vi "fifo configure (host).vi"(8 "error in":errorcluster, 11 "niUsrpRio Session (in)":T1 {"Daughterboard Clock Rate" format="%#.3pHz"; "FPGA Data Clock Rate" format="%#.3pHz"; "Data Clock Rate" format="%#.3pHz"; "Characterization Data"."Frequencies [Hz]" format="%#_6p"; "EEPROM Characterization Header"."Pointer to Device Data Header" format="%x"; "EEPROM Characterization Header"."Checksum" format="%x"; "Device Data Header"."Pointer to Characterization Data" format="%x"; "Device Data Header"."Checksum" format="%x"; "EEPROM Header"."Pointer to User Header" format="%x"; "EEPROM Header"."Pointer to Factory Header" format="%x"; "EEPROM Header"."Product Code" format="%x"; "EEPROM Header"."Checksum" format="%x"}) -> (0 "error out":errorcluster, 3 "niUsrpRio Session (out)":T1 {"Daughterboard Clock Rate" format="%#.3pHz"; "FPGA Data Clock Rate" format="%#.3pHz"; "Data Clock Rate" format="%#.3pHz"; "Characterization Data"."Frequencies [Hz]" format="%#_6p"; "EEPROM Characterization Header"."Pointer to Device Data Header" format="%x"; "EEPROM Characterization Header"."Checksum" format="%x"; "Device Data Header"."Pointer to Characterization Data" format="%x"; "Device Data Header"."Checksum" format="%x"; "EEPROM Header"."Pointer to User Header" format="%x"; "EEPROM Header"."Pointer to Factory Header" format="%x"; "EEPROM Header"."Product Code" format="%x"; "EEPROM Header"."Checksum" format="%x"})   [LabVIEW 2020]
uses:
  <instrlib>/niUsrpRio/Config/v1/Host/Public/niUsrpRio Session.ctl
  <instrlib>/_niInstr/Register Bus/v0/Host/Public/Register Bus Session.ctl
  <instrlib>/_niInstr/Register Bus/v0/Host/Private/Session Data.ctl
  <instrlib>/niUsrpRio/Config/v1/Host/Private/DB Queue Reference.ctl
  <instrlib>/niUsrpRio/Config/v1/Host/Private/Daughterboard Data.ctl
  <instrlib>/niUsrpRio/Config/v1/Host/Private/ATR state data.ctl
  <instrlib>/niUsrpRio/Config/v1/Host/Private/Antenna Configuration.ctl
  <instrlib>/niUsrpRio/Config/v1/Host/Private/CPLD Power Mode.ctl
  <instrlib>/niUsrpRio/Config/v1/Host/Public/EEPROM Header.ctl
  <instrlib>/niUsrpRio/Config/v1/Host/Public/EEPROM Device Data Header.ctl
  <instrlib>/niUsrpRio/Config/v1/Host/Public/EEPROM Characterization Header.ctl
  <instrlib>/niUsrpRio/Config/v1/Host/Public/Characterization Data.ctl
  <instrlib>/niUsrpRio/Config/v1/Host/Public/IQ Imbalance.ctl
  Host/SubVIs/Streaming Xvcr FPGA Ref.ctl
  <vilib>/Utility/error.llb/Error Cluster From Error Code.vi
  <vilib>/rvi/interface/common/niFpgaWaitOnOcc.vi
  <vilib>/rvi/interface/nirviMethod/nirviMethod.xnode
  <vilib>/FPGAPlugInAG/Dynamic/niLvFpga_ConfigureFifo_Dynamic.vi
  <vilib>/rvi/errors/niLvFpgaMergeErrorWithErrorCode.vi
  <vilib>/FPGAPlugInAG/Dynamic/niLvFpga_StopFifo_Dynamic.vi
  <vilib>/FPGAPlugInAG/Dynamic/niLvFpga_StartFifo_Dynamic.vi
  <instrlib>/_niInstr/Register Bus/v0/Host/niInstr Register Bus v0 Host.lvlib
  <instrlib>/niUsrpRio/Config/v1/Host/niUsrpRio Config v1 Host.lvlib
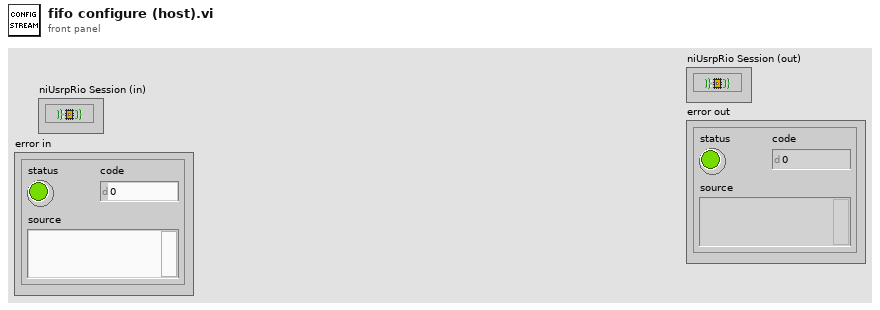
[diagram p1: front panel]
types:
  T1 = typedef "niUsrpRio Config v1 Host.lvlib/niUsrpRio Session.ctl" = cluster{"FPGA Interface":refnum<k20>, "RIO Interface Number":u32, "Data Clock Rate":u32, "FPGA Data Clock Rate":u32, "Global Settings Register Bus":T2, "Radio 0 Settings Register Bus":T2, "Radio 1 Settings Register Bus":T2, "Radio Settings Bus Semaphore":T3, "DB Queues":T4[], "Characterization Data Valid?":bool, "EEPROM Header":T5, "Device Data Header":T6, "EEPROM Characterization Header":T7, "Characterization Data":T8[], "FPGA Current Version":u32, "FPGA Oldest Compatible Version":u32, "Fixed Logic Current Version":u32, "Fixed Logic Oldest Compatible Version":u32, "FPGA Radio Settings Bus Current Version":u32, "FPGA Radio Settings Bus Oldest Compatible Version":u32, "FPGA Board Config Current Version":u32, "FPGA Board Config Oldest Compatible Version":u32, "Daughterboard Clock Rate":u32, "daughterboard configuration session handles":u64[]}
  T2 = typedef "niInstr Register Bus v0 Host.lvlib/Register Bus Session.ctl" = refnum<queue>
  T3 = typedef "Semaphore RefNum" = refnum<k1>
  T4 = typedef "niUsrpRio Config v1 Host.lvlib/DB Queue Reference.ctl" = refnum<queue>
  T5 = typedef "niUsrpRio Config v1 Host.lvlib/EEPROM Header.ctl" = cluster{"Checksum":u32, "Product Code":u16, "Hardware Current Version":u16, "Hardware Oldest Compatible Version":u16, "EEPROM Map Current Version":u16, "EEPROM Map Oldest Compatible Version":u16, "User Password":string, "Pointer to Factory Header":u32, "Pointer to User Header":u32, "Recommended Interval":u16, "Number of Reserved Bytes":i32, "Number of Daughterboards":u8, "Daughterboard IDs":u16[], "Daughterboard Serial Numbers":string[]}
  T6 = typedef "niUsrpRio Config v1 Host.lvlib/EEPROM Device Data Header.ctl" = cluster{"Checksum":u32, "Number of Channels":u8, "Number of Gain Settings":u16[], "Pointer to Characterization Data":u32[], "Number of Reserved Bytes":i32, "Number of Frequencies":u16[]}
  T7 = typedef "niUsrpRio Config v1 Host.lvlib/EEPROM Characterization Header.ctl" = cluster{"Checksum":u32, "Date":timestamp, "Temperature":sgl, "Misc. Info":string, "Pointer to Device Data Header":u32, "Number of Reserved Bytes":i32}
  T8 = typedef "niUsrpRio Config v1 Host.lvlib/Characterization Data.ctl" = cluster{"Gains[dB]":dbl[], "Frequencies [Hz]":dbl[], "IQ Imbalance Table":T9[], "Measured Gains[dB]":dbl[][]}
  T9 = typedef "niUsrpRio Config v1 Host.lvlib/IQ Imbalance.ctl" = cluster{"Gain Imbalance [linear]":dbl, "Phase Imbalance [radians]":dbl, "Offset":cdb}
  T10 = typedef "Streaming Xvcr FPGA Ref.ctl" = refnum<k20>
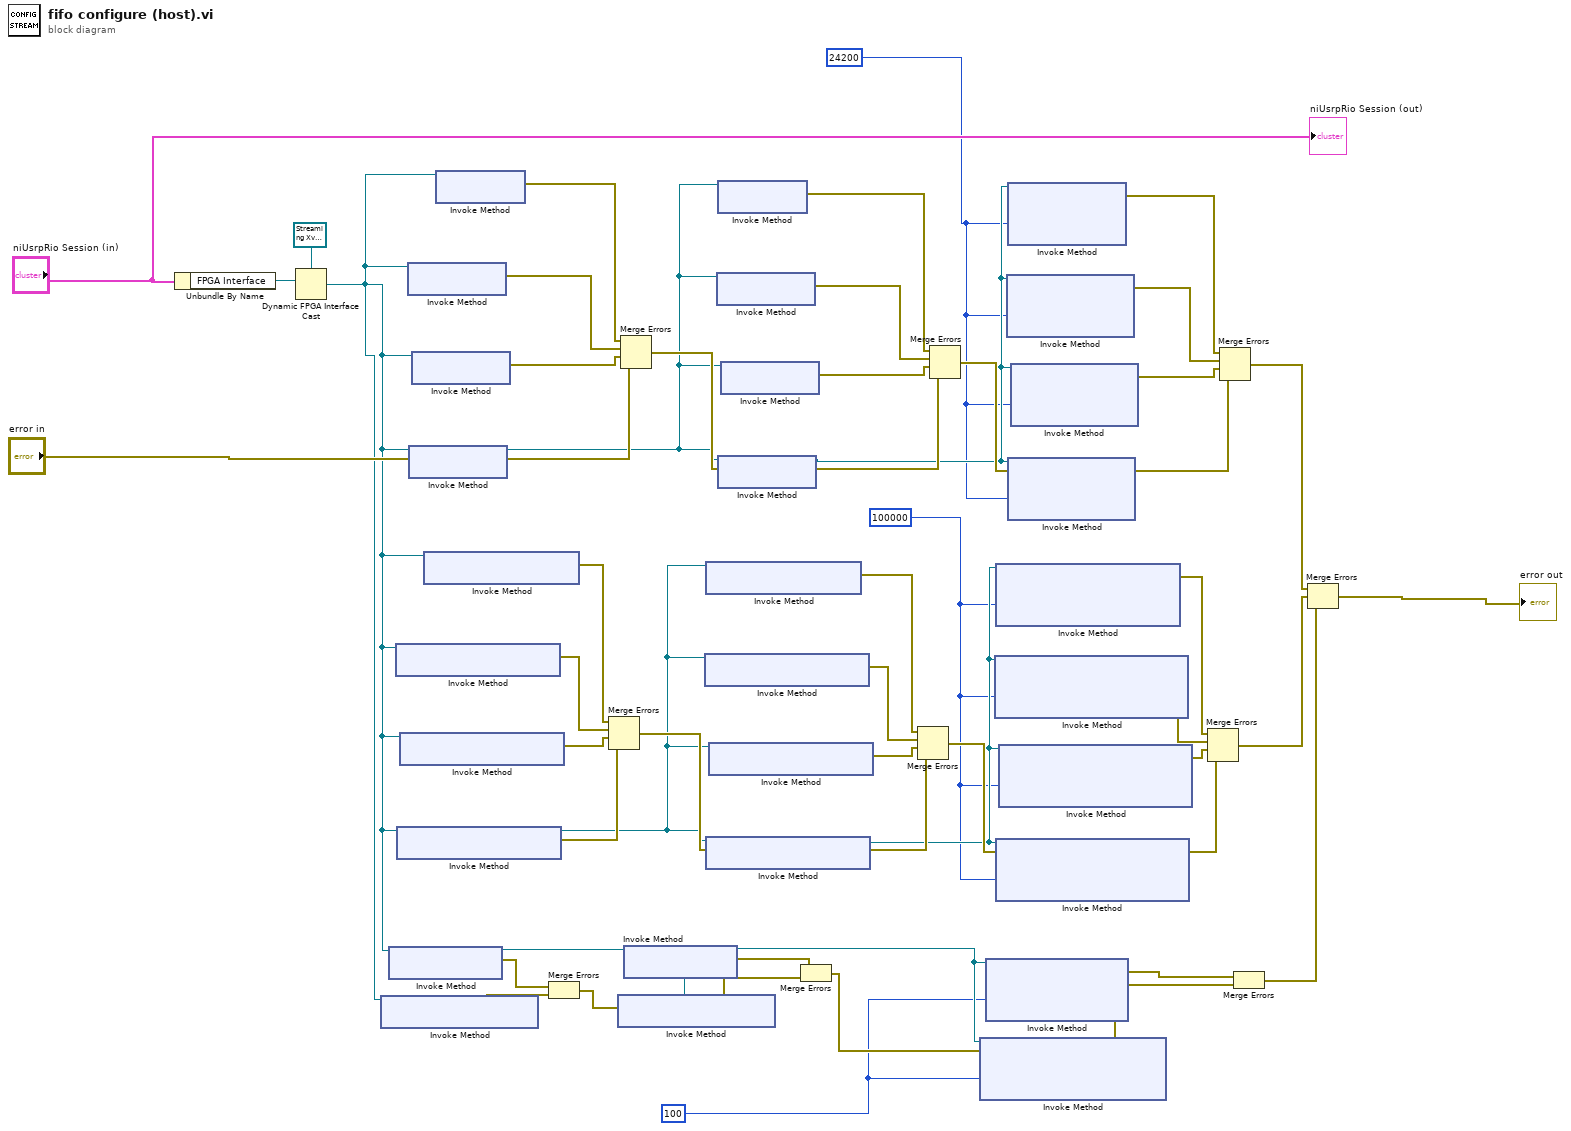
[diagram p0: block diagram]
diagram:
  w1 = u32 100000 ("Requested Depth")
  w2 = u32 24200 ("Requested Depth")
  w3 = u32 100 ("Requested Depth")
  n1 = Unbundle By Name("niUsrpRio Session (in)") -> ("FPGA Interface"=w53:refnum<k20>)
  n2 = Dynamic FPGA Interface Cast(Session In=T10 refnum ("Type"), Type=w53) -> (Session Out=w10:T10)
  n3 = xnode "Invoke Method"("FPGA VI Reference In"=w10) -> ("error out"=w15:errorcluster)  [unwired: 1 in, 1 out]
  n4 = xnode "Invoke Method"("FPGA VI Reference In"=w10) -> ("FPGA VI Reference Out"=w9:T10, "error out"=w16:errorcluster)  [unwired: 1 in]
  n5 = xnode "Invoke Method"("FPGA VI Reference In"=w10) -> ("error out"=w31:errorcluster)  [unwired: 1 in, 1 out]
  n6 = xnode "Invoke Method"("FPGA VI Reference In"=w10) -> ("FPGA VI Reference Out"=w19:T10, "error out"=w29:errorcluster)  [unwired: 1 in]
  n7 = xnode "Invoke Method"("FPGA VI Reference In"=w10) -> ("error out"=w30:errorcluster)  [unwired: 1 in, 1 out]
  n8 = xnode "Invoke Method"("FPGA VI Reference In"=w10) -> ("error out"=w50:errorcluster)  [unwired: 1 in, 1 out]
  n9 = xnode "Invoke Method"("FPGA VI Reference In"=w10, "error in"="error in") -> ("FPGA VI Reference Out"=w38:T10, "error out"=w48:errorcluster)
  n10 = xnode "Invoke Method"("FPGA VI Reference In"=w10) -> ("error out"=w49:errorcluster)  [unwired: 1 in, 1 out]
  n11 = xnode "Invoke Method"("FPGA VI Reference In"=w10) -> ("error out"=w32:errorcluster)  [unwired: 1 in, 1 out]
  n12 = xnode "Invoke Method"("FPGA VI Reference In"=w10) -> ("error out"=w51:errorcluster)  [unwired: 1 in, 1 out]
  n13 = Merge Errors(w16, w15) -> (w7:errorcluster)
  n14 = Merge Errors(w32, w31, w30, w29) -> (w20:errorcluster)
  n15 = xnode "Invoke Method"("FPGA VI Reference In"=w9, "error in"=w7) -> ("error out"=w13:errorcluster)  [unwired: 1 out]
  n16 = Merge Errors(w51, w50, w49, w48) -> (w39:errorcluster)
  n17 = xnode "Invoke Method"("FPGA VI Reference In"=w9) -> ("FPGA VI Reference Out"=w8:T10, "error out"=w14:errorcluster)  [unwired: 1 in]
  n18 = xnode "Invoke Method"("FPGA VI Reference In"=w19) -> ("error out"=w27:errorcluster)  [unwired: 1 in, 1 out]
  n19 = xnode "Invoke Method"("FPGA VI Reference In"=w19) -> ("error out"=w28:errorcluster)  [unwired: 1 in, 1 out]
  n20 = xnode "Invoke Method"("FPGA VI Reference In"=w19, "error in"=w20) -> ("FPGA VI Reference Out"=w17:T10, "error out"=w25:errorcluster)
  n21 = xnode "Invoke Method"("FPGA VI Reference In"=w19) -> ("error out"=w26:errorcluster)  [unwired: 1 in, 1 out]
  n22 = xnode "Invoke Method"("FPGA VI Reference In"=w38) -> ("error out"=w46:errorcluster)  [unwired: 1 in, 1 out]
  n23 = xnode "Invoke Method"("FPGA VI Reference In"=w38) -> ("error out"=w47:errorcluster)  [unwired: 1 in, 1 out]
  n24 = xnode "Invoke Method"("FPGA VI Reference In"=w38, "error in"=w39) -> ("FPGA VI Reference Out"=w36:T10, "error out"=w44:errorcluster)
  n25 = xnode "Invoke Method"("FPGA VI Reference In"=w38) -> ("error out"=w45:errorcluster)  [unwired: 1 in, 1 out]
  n26 = Merge Errors(w14, w13) -> (w6:errorcluster)
  n27 = Merge Errors(w28, w27, w26, w25) -> (w18:errorcluster)
  n28 = Merge Errors(w47, w46, w45, w44) -> (w37:errorcluster)
  n29 = xnode "Invoke Method"("FPGA VI Reference In"=w8, "error in"=w6, "Requested Depth"=w3) -> ("error out"=w11:errorcluster)  [unwired: 2 out]
  n30 = xnode "Invoke Method"("FPGA VI Reference In"=w8, "Requested Depth"=w3) -> ("error out"=w12:errorcluster)  [unwired: 1 in, 2 out]
  n31 = xnode "Invoke Method"("FPGA VI Reference In"=w17, "Requested Depth"=w1) -> ("error out"=w23:errorcluster)  [unwired: 1 in, 2 out]
  n32 = xnode "Invoke Method"("FPGA VI Reference In"=w17, "Requested Depth"=w1) -> ("error out"=w24:errorcluster)  [unwired: 1 in, 2 out]
  n33 = xnode "Invoke Method"("FPGA VI Reference In"=w17, "error in"=w18, "Requested Depth"=w1) -> ("error out"=w21:errorcluster)  [unwired: 2 out]
  n34 = xnode "Invoke Method"("FPGA VI Reference In"=w17, "Requested Depth"=w1) -> ("error out"=w22:errorcluster)  [unwired: 1 in, 2 out]
  n35 = xnode "Invoke Method"("FPGA VI Reference In"=w36, "Requested Depth"=w2) -> ("error out"=w42:errorcluster)  [unwired: 1 in, 2 out]
  n36 = xnode "Invoke Method"("FPGA VI Reference In"=w36, "Requested Depth"=w2) -> ("error out"=w43:errorcluster)  [unwired: 1 in, 2 out]
  n37 = xnode "Invoke Method"("FPGA VI Reference In"=w36, "error in"=w37, "Requested Depth"=w2) -> ("error out"=w40:errorcluster)  [unwired: 2 out]
  n38 = xnode "Invoke Method"("FPGA VI Reference In"=w36, "Requested Depth"=w2) -> ("error out"=w41:errorcluster)  [unwired: 1 in, 2 out]
  n39 = Merge Errors(w24, w23, w22, w21) -> (w5:errorcluster)
  n40 = Merge Errors(w43, w42, w41, w40) -> (w35:errorcluster)
  n41 = Merge Errors(w12, w11) -> (w4:errorcluster)
  n42 = Merge Errors(w35, w5, w4) -> (→"error out":errorcluster)
  "niUsrpRio Session (out)" <- "niUsrpRio Session (in)"
